vi "Get System Environment Variable.vi"(3 "Environment Variable Name":string="COMPUTERNAME") -> (1 "Value":string)   [LabVIEW 2017]
doc: "Reads the value of the named Windows environment variable."
uses:
  kernel32.dll
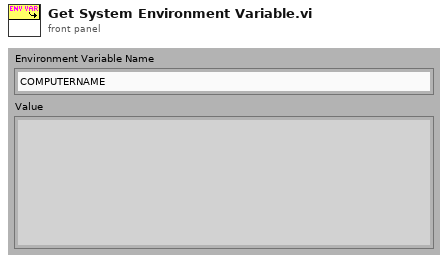
[diagram p1: front panel]
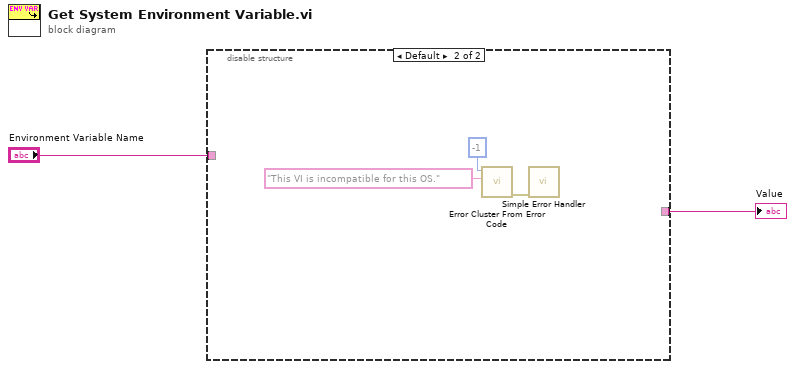
[diagram p0: block diagram]
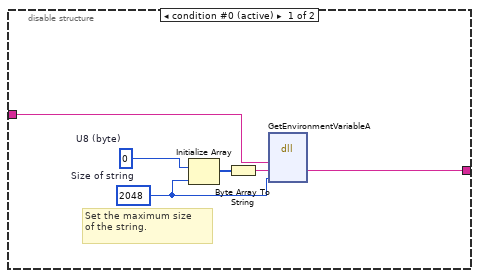
[diagram p2: hidden frame]
diagram:
  n1 = disable-structure shown="Default" {
    disable-tunnel: "Environment Variable Name" -> [w8 _]
    disable-tunnel: [w7 _] -> w1
    frame condition #0 (active) {
      w5 = u8 0  # U8 (byte)
      w6 = 2048  # Size of string
      # "Set the maximum size\nof the string."
      n2 = Initialize Array(w5, w6) -> (w4:u8[])
      n3 = Byte Array To String(unsigned byte array=w4) -> (string=w3:string)
      n4 = dll-call lib="kernel32.dll" fn="GetEnvironmentVariableA"("EnvVarName"=w8, "lpBuffer"=w3, "namelength"=w6) -> ("lpBuffer"=w7:string)  [unwired: 6 in, 2 out]
    }
    frame condition #1 {
      n5 = call <vilib>:"Error Cluster From Error Code.vi"("error message (\"\")"="This VI is incompatible for this OS." ("error message (\"\")"), "error code (0)"=-1) -> ("error out"=w9:errorcluster)  [unwired: 7 in]
      n6 = call <vilib>:"Simple Error Handler.vi"("error in (no error)"=w9) -> ()  [unwired: 4 in, 5 out]
    }
  }
  "Value" <- w1
